vi "testbufferrollover_wfmmap.vi"() -> ()   [LabVIEW 2017]
uses:
  <vilib>/addons/InsightCM/Devices/Shared/Common/DataFlow/controls/Data.ctl
  <vilib>/addons/InsightCM/Utilities/DataAccessors/controls/wfmSGL_DVR.ctl
  <vilib>/addons/PointValueMap/controls/PointMap.ctl
  <vilib>/addons/InsightCM/Devices/Shared/Common/DataFlow/controls/Type.ctl
  <vilib>/addons/PointValueMap/subVIs/Point_Write_i32.vi
  <vilib>/addons/InsightCM/Devices/Shared/Common/DVRBuffer/DVRBuffer.lvlib
  <vilib>/addons/PointValueMap/PointValueMap.lvlib
  <vilib>/addons/InsightCM/Devices/Shared/Common/DataFlow/DataFlow.lvlib
  <vilib>/measure/NI_MABase.lvlib
panel:
  out "Waveform Graph":waveform(sgl)[](graph)
  out "logical AND":bool
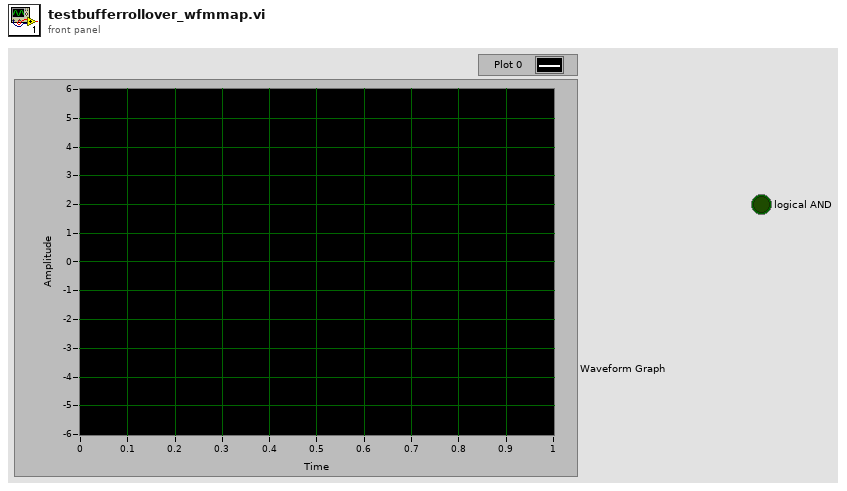
[diagram p1: front panel]
types:
  T1 = typedef "DataFlow.lvlib/Data.ctl" = cluster{"DataGroup":string, "Waveforms":T2, "Map":T3, "Type":T4}
  T2 = typedef "wfmSGL_DVR.ctl" = refnum<data-value>
  T3 = typedef "PointValueMap.lvlib/PointMap.ctl" = refnum<data-value>
  T4 = typedef "DataFlow.lvlib/Type.ctl" = enum16{"High Rate", "Low Rate", "Burst Mode"}
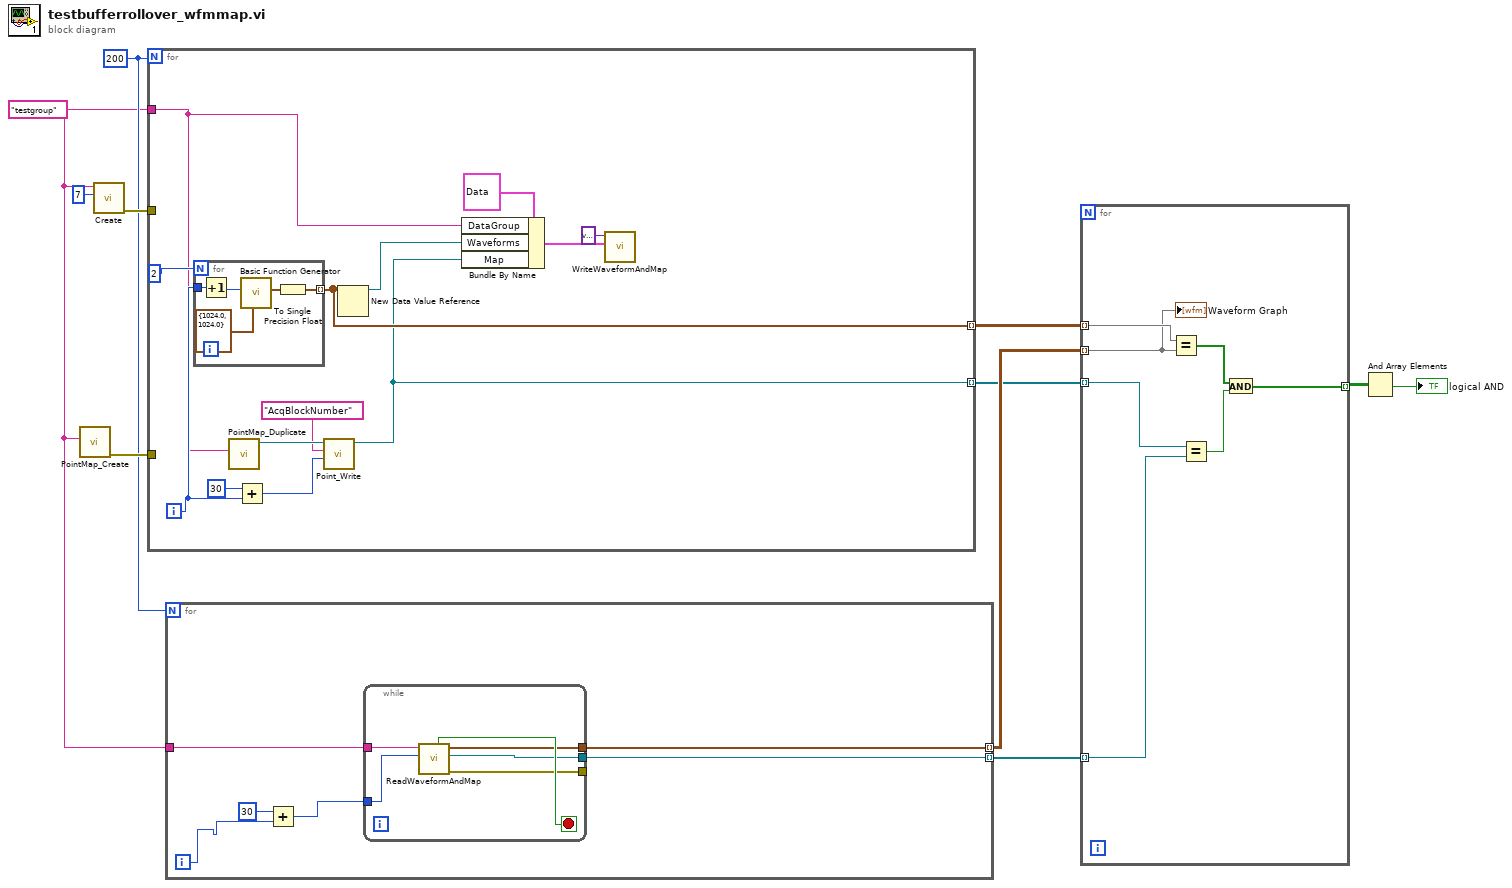
[diagram p0: block diagram]
diagram:
  w8 = 200
  w7 = "testgroup" ("name")
  n1 = call <vilib>:"PointMap_Create.vi"("Name"=w7) -> ("error out"=w9:errorcluster)  [unwired: 9 in, 1 out]
  n2 = call <vilib>:"Create.vi"("size"=7, "name"=w7) -> ("error out"=w10:errorcluster)  [unwired: 8 in, 1 out]
  n3 = for {
    N: w8 -> [_]
    tunnel: w7 -> [w14]
    tunnel: w10 -> [_]
    tunnel: w9 -> [_]
    tunnel: [w13] -> w5 mode=indexing
    tunnel: [w12] -> w4 mode=indexing
    i -> [w17]
    n4 = for {
      N: 2 -> [_]
      tunnel: [w27] -> w13 mode=indexing
      tunnel: w17 -> [w25]
      n5 = Increment(x=w25) -> (x+1=w26:i32)
      n6 = call <vilib>:"Basic Function Generator.vi"("sampling info"=cluster{"Fs":dbl, "#s":dbl} {"Fs"=1024.0, "#s"=1024.0}, "amplitude"=w26) -> ("signal out"=w28:waveform(dbl))  [unwired: 7 in, 2 out]
      n7 = To Single Precision Float(number=w28) -> (single precision float=w27:waveform(sgl))
    }
    n8 = call <vilib>:"PointMap_Duplicate.vi"("Source Map Name"=w14) -> ("Map Out"=w19:T3)  [unwired: 9 in, 1 out]
    n9 = Add(x=30, y=w17) -> (x+y=w15:i32)
    n10 = call-poly <vilib>:"Point_Write.vi"("Value"=w15, "Tag"="AcqBlockNumber", "Map"=w19) -> ("Map Out"=w12:T3)  [unwired: 7 in, 1 out]
    n11 = New Data Value Reference(data value=w13) -> (data value reference=w22:refnum<data-value>)  [unwired: 1 in, 1 out]
    n12 = Bundle By Name(cluster=T1 {"DataGroup"="", "Waveforms"=refnum, "Map"=refnum, "Type"=enum."High Rate"} ("data"), "DataGroup"=w14, "Waveforms"=w22, "Map"=w12) -> (w21:T1)
    n13 = call <vilib>:"WriteWaveformAndMap.vi"("data"=w21, "config"=variant) -> ()  [unwired: 7 in, 3 out]
  }
  n14 = for {
    N: w8 -> [_]
    tunnel: w7 -> [w35]
    tunnel: [w34] -> w6 mode=indexing
    tunnel: [w33] -> w3 mode=indexing
    i -> [w31]
    n15 = Add(x=30, y=w31) -> (x+y=w30:i32)
    n16 = while {
      tunnel: w35 -> [w41]
      tunnel: [w39] -> w34
      tunnel: [w38] -> w33
      tunnel: w30 -> [w37]
      tunnel: [w36] -> _
      stop <- w40 stop-if-true
      n17 = call <vilib>:"ReadWaveformAndMap.vi"("buffer location"=w37, "data group"=w41) -> ("error out"=w36:errorcluster, "map"=w38:T3, "waveforms"=w39:waveform(sgl)[], "found"=w40:bool)  [unwired: 5 in, 1 out]
    }
  }
  n18 = for {
    tunnel: w6 -> [w42] mode=indexing
    tunnel: w5 -> [w48] mode=indexing
    tunnel: w4 -> [w47] mode=indexing
    tunnel: w3 -> [w46] mode=indexing
    tunnel: [w43] -> w2 mode=indexing
    n19 = Equal?(x=w48, y=w42) -> (x = y?=w45:bool[])
    n20 = Equal?(x=w47, y=w46) -> (x = y?=w44:bool)
    n21 = And(x=w45, y=w44) -> (x .and. y?=w43:bool[])
    "Waveform Graph" <- w42
  }
  n22 = And Array Elements(Boolean array=w2) -> (logical AND=→"logical AND":bool)
